vi "Actor Core.vi"(8 "error in":errorcluster caption="错误输入", 11 "硬件代理者 in":refnum<class "硬件代理者.lvclass"> caption="操作者输入") -> (0 "error out":errorcluster caption="错误输出", 3 "Actor out":refnum<class "Actor.lvclass"> caption="操作者输出")   [LabVIEW 2015, in "硬件代理者.lvlib" / "硬件代理者.lvclass"]
doc: "(<B>文件名</B>: Actor Framework.lvlib:Actor.lvclass:Actor Core.vi)\n\n接收发送至操作者的消息，响应消息并处理可能导致操作者关闭的错误。\n\n子孙类重写该VI，使操作者完成特定的任务。使用调用父方法节点实现重写。"
uses:
  <vilib>/ActorFramework/Actor/Actor.lvclass
panel:
  out "已经发送":string
  out "已收到":string
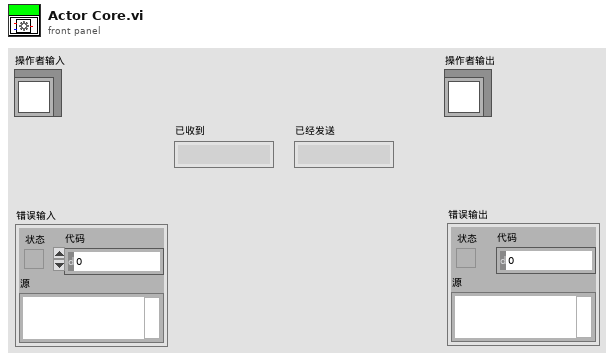
[diagram p1: front panel]
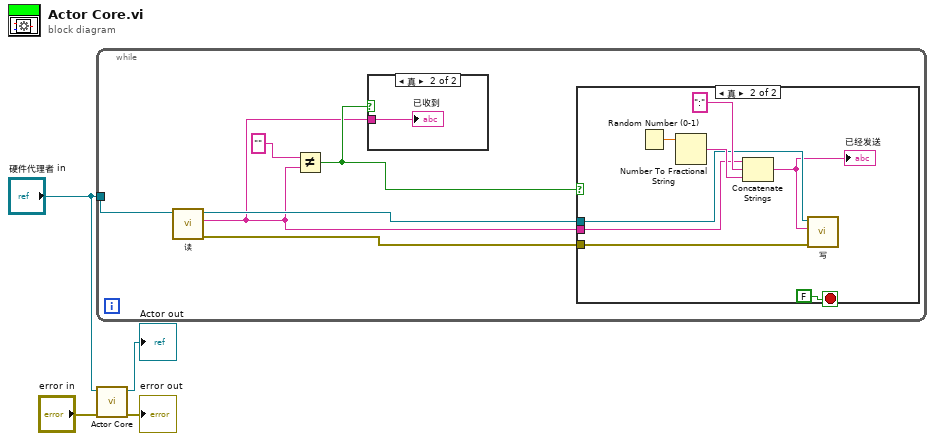
[diagram p0: block diagram]
diagram:
  n1 = while {
    tunnel: "硬件代理者 in" -> [w10]
    stop <- FALSE stop-if-true
    n2 = call-dynamic "读.vi"("通讯 输入"=w10) -> ("error out"=w8:errorcluster, "读取缓冲区"=w5:string, "通讯 输出"=w9:refnum<class "硬件代理者.lvclass">)  [unwired: 8 in]
    n3 = Not Equal?(x="", y=w5) -> (x != y?=w6:bool)
    n4 = case shown="真" w6 {
      tunnel: w5 -> [_ w12]
      frame False {
      }
      frame True {
        "已收到" <- w12
      }
    }
    n5 = case shown="真" w6 {
      tunnel: w5 -> [_ w16]
      tunnel: w9 -> [_ w15]
      tunnel: w8 -> [_ w13]
      frame False {
      }
      frame True {
        n6 = Random Number (0-1)() -> (number: 0 to 1=w19:dbl)
        n7 = Number To Fractional String(number=w19) -> (F-format string=w17:string)  [unwired: 3 in]
        n8 = Concatenate Strings(w16, ":", w17) -> (w14:string)
        "已经发送" <- w14
        n9 = call-dynamic "写.vi"("error in (no error)"=w13, "写入缓冲区"=w14, "通讯 输入"=w15) -> ()  [unwired: 7 in, 2 out]
      }
    }
  }
  n10 = call-parent "Actor Core.vi"("error in"="error in", "Actor in"="硬件代理者 in") -> ("error out"=→"error out":errorcluster, "Actor out"=→"Actor out":refnum<class "Actor.lvclass">)  [unwired: 8 in]
